vi "gen_shift_curr_pattern.vi"(0 "Cycles per readout":dbl=250.0, 5 "Waveform type":enum16{"None", "Stair", "Ramp", "Sine"}(ring)=enum."Stair", 7 "Readouts per projection":i32=10, 9 "Ramp start":dbl=1.0, 11 "Ramp stop":dbl=-1.0, 12 "Ramp-up readouts":i32=250, 13 "Wait readouts":i32) -> (4 "output waveform":waveform(dbl)={"t0"=timestamp(0 s since 1904-01-01), "dt"=1.0, "Y"=array[60000 elements]}, 15 "waveform length":i32)   [LabVIEW 2019]
uses:
  <vilib>/Analysis/1siggen.llb/Ramp Pattern by Samples.vi
  global_variables.vi
  <vilib>/Analysis/NI_AALBase.lvlib
panel:
  out "Waveform Graph":waveform(dbl)(graph)={"t0"=timestamp(0 s since 1904-01-01), "dt"=1.0, "Y"=array[60000 elements]}
  out "Sample points per TX cycle":dbl=20.0
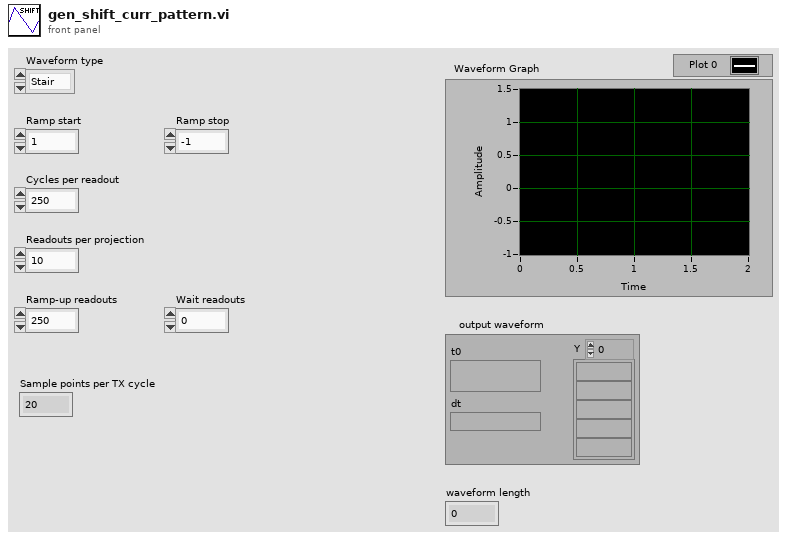
[diagram p1: front panel]
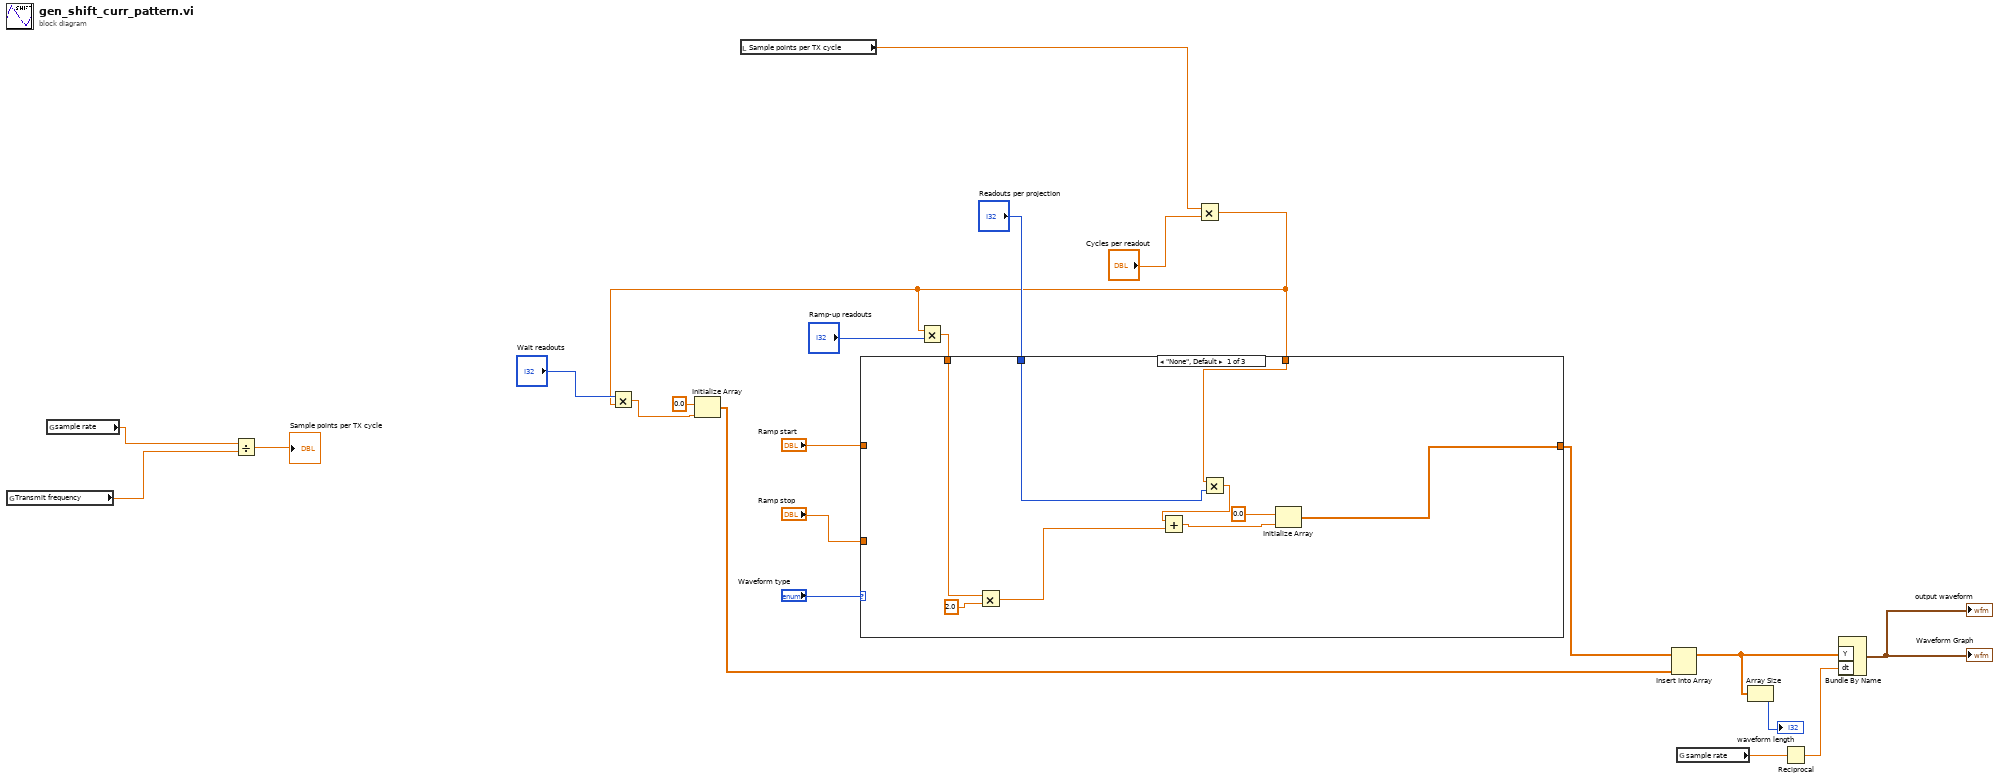
[diagram p0: block diagram]
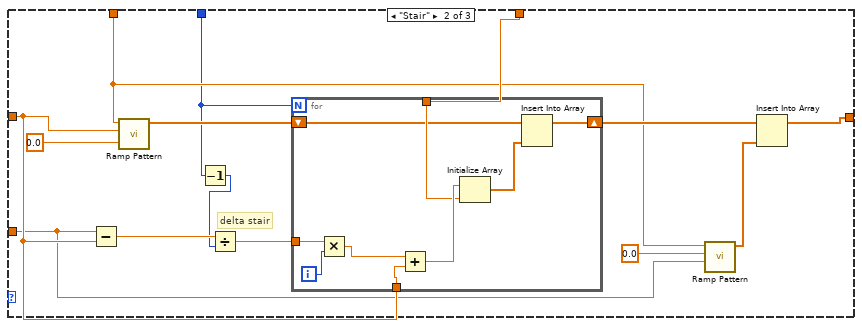
[diagram p2: hidden frame]
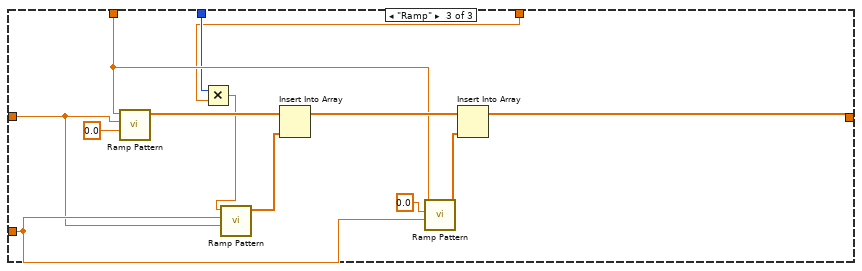
[diagram p3: hidden frame]
diagram:
  n1 = global read "global_variables.vi" "Transmit frequency"() -> (w7:dbl)
  n2 = global read "global_variables.vi" "sample rate"() -> (w6:dbl)
  n3 = Divide(x=w6, y=w7) -> (x/y=→"Sample points per TX cycle":dbl)
  n4 = local read "Sample points per TX cycle"() -> (w13:dbl)
  n5 = Multiply(x=w13, y="Cycles per readout") -> (x*y=w8:dbl)
  n6 = Multiply(x="Wait readouts", y=w8) -> (x*y=w18:dbl)
  n7 = Initialize Array(0.0 ("element"), w18) -> (w10:dbl[])
  n8 = Multiply(x=w8, y="Ramp-up readouts") -> (x*y=w12:dbl)
  n9 = case shown="\"None\", Default" "Waveform type" {
    tunnel: [w28 w34 w63] -> w1
    tunnel: "Ramp start" -> [_ w42 w58]
    tunnel: "Ramp stop" -> [_ w35 w59]
    tunnel: w12 -> [w27 w37 w60]
    tunnel: w8 -> [w26 w40 w56]
    tunnel: "Readouts per projection" -> [w25 w32 w57]
    frame "None", Default {
      n10 = Multiply(x=w27, y=2.0) -> (x*y=w30:dbl)
      n11 = Multiply(x=w26, y=w25) -> (x*y=w24:dbl)
      n12 = Add(x=w24, y=w30) -> (x+y=w23:dbl)
      n13 = Initialize Array(0.0 ("element"), w23) -> (w28:dbl[])
    }
    frame "Stair" {
      # "delta stair"
      n14 = Subtract(x=w35, y=w42) -> (x-y=w43:dbl)
      n15 = call-poly <vilib>:"Ramp Pattern.vi"("start"=0.0, "end"=w42, "samples"=w37) -> ("Ramp Pattern"=w44:dbl[])  [unwired: 7 in, 1 out]
      n16 = Decrement(x=w32) -> (x-1=w33:i32)
      n17 = Divide(x=w43, y=w33) -> (x/y=w41:dbl)
      n18 = for {
        N: w32 -> [_]
        shift-right: [w46] -> w39
        shift-left: w44 -> [w48]
        tunnel: w42 -> [w54]
        tunnel: w41 -> [w53]
        tunnel: w40 -> [w49]
        i -> [w52]
        n19 = Multiply(x=w53, y=w52) -> (x*y=w51:dbl)
        n20 = Add(x=w51, y=w54) -> (x+y=w50:dbl)
        n21 = Initialize Array(w50, w49) -> (w47:dbl[])
        n22 = Insert Into Array(array=w48, new element=w47) -> (w46:dbl[])  [unwired: 1 in]
      }
      n23 = call-poly <vilib>:"Ramp Pattern.vi"("start"=w35, "end"=0.0, "samples"=w37) -> ("Ramp Pattern"=w38:dbl[])  [unwired: 7 in, 1 out]
      n24 = Insert Into Array(array=w39, new element=w38) -> (w34:dbl[])  [unwired: 1 in]
    }
    frame "Ramp" {
      n25 = call-poly <vilib>:"Ramp Pattern.vi"("start"=0.0 ("end"), "end"=w58, "samples"=w60) -> ("Ramp Pattern"=w66:dbl[])  [unwired: 7 in, 1 out]
      n26 = Multiply(x=w57, y=w56) -> (x*y=w55:dbl)
      n27 = call-poly <vilib>:"Ramp Pattern.vi"("start"=w58, "end"=w59, "samples"=w55) -> ("Ramp Pattern"=w65:dbl[])  [unwired: 7 in, 1 out]
      n28 = Insert Into Array(array=w66, new element=w65) -> (w64:dbl[])  [unwired: 1 in]
      n29 = call-poly <vilib>:"Ramp Pattern.vi"("start"=w59, "end"=0.0, "samples"=w60) -> ("Ramp Pattern"=w62:dbl[])  [unwired: 7 in, 1 out]
      n30 = Insert Into Array(array=w64, new element=w62) -> (w63:dbl[])  [unwired: 1 in]
    }
  }
  n31 = Insert Into Array(array=w1, new element=w10) -> (w2:dbl[])  [unwired: 1 in]
  n32 = global read "global_variables.vi" "sample rate"() -> (w5:dbl)
  n33 = Array Size(array=w2) -> (size(s)=→"waveform length":i32)
  n34 = Reciprocal(x=w5) -> (1/x=w3:dbl)
  n35 = Bundle By Name("Y"=w2, "dt"=w3) -> (→"Waveform Graph" →"output waveform":waveform(dbl))  [unwired: 1 in]
